vi "图形控件之XY图的使用.vi"() -> ()   [LabVIEW 2018]
panel:
  out "XY Graph":cluster{"Y":dbl[], "Y":dbl[]}[](graph) caption="XY图"
  out "XY图 2":cluster{dbl[], dbl[]}(graph)
  out "XY图":cluster{dbl, dbl, dbl}[](graph)
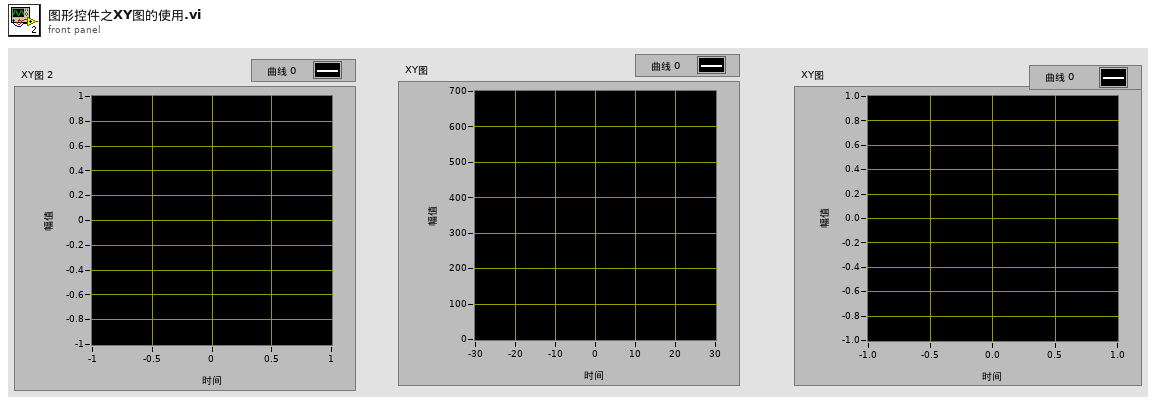
[diagram p1: front panel]
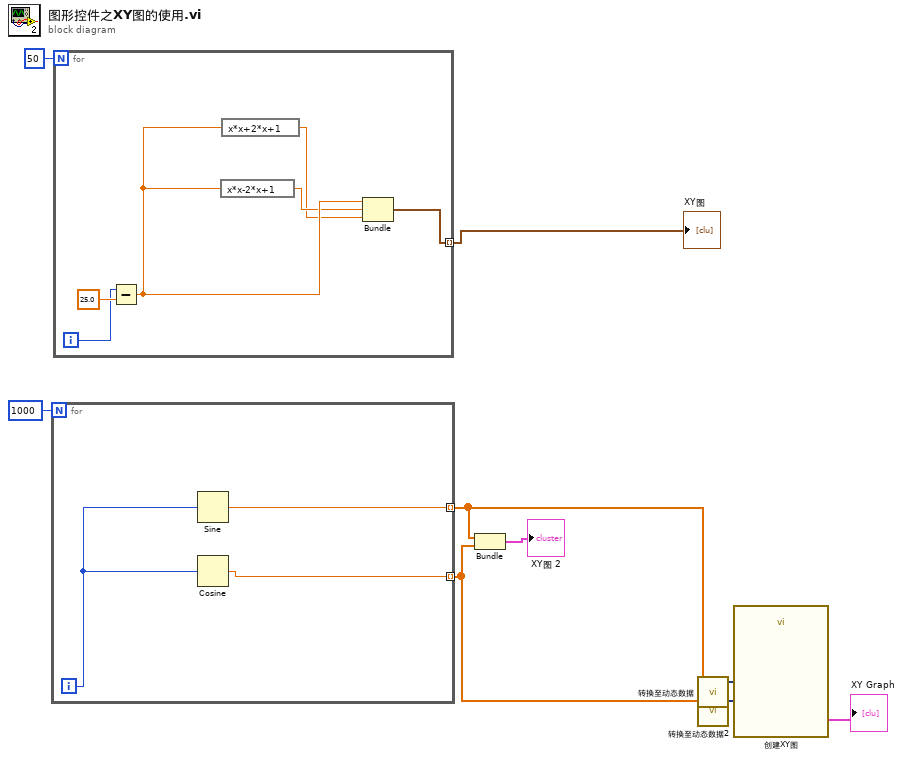
[diagram p0: block diagram]
diagram:
  n1 = for {
    N: 1000 -> [_]
    tunnel: [w11] -> w4 mode=indexing
    tunnel: [w10] -> w2 mode=indexing
    i -> [w12]
    n2 = Sine(x=w12) -> (sin(x)=w11:dbl)
    n3 = Cosine(x=w12) -> (cos(x)=w10:dbl)
  }
  n4 = for {
    N: 50 -> [_]
    tunnel: [w13] -> w8 mode=indexing
    i -> [w17]
    n5 = Subtract(x=w17, y=25.0) -> (x-y=w16:dbl)
    n6 = expression code="x*x-2*x+1"(w16) -> (w15:dbl)
    n7 = expression code="x*x+2*x+1"(w16) -> (w14:dbl)
    n8 = Bundle(w16, w15, w14) -> (w13:cluster{dbl, dbl, dbl})  [unwired: 1 in]
  }
  "XY图" <- w8
  n9 = Bundle(w4, w2) -> (→"XY图 2":cluster{dbl[], dbl[]})  [unwired: 1 in]
  n10 = call "转换至动态数据"("Array"=w4) -> ("Dynamic Data Type"=w3:dynamicdata)  [unwired: 3 in]
  n11 = call "转换至动态数据2"("Array"=w2) -> ("Dynamic Data Type"=w1:dynamicdata)  [unwired: 3 in]
  n12 = call "创建XY图"("Y Input"=w1, "X Input"=w3) -> ("XY Graph"=→"XY Graph":cluster{"X":dbl[], "Y":dbl[]}[])  [unwired: 8 in, 1 out]
